vi "Prime calculator.vi"(6 "IR":dbl, 8 "Blue":i16, 9 "Green":i16, 10 "Red":i16, 11 "Clear":i16) -> (0 "B'":dbl, 1 "G'":dbl, 2 "R'":dbl, 3 "C'":dbl)   [LabVIEW 2016, in "AMS TS3472 Light Sensor.lvlib" / "AMS TCS3472.lvclass"]
uses:
  AMS TCS3472.lvclass
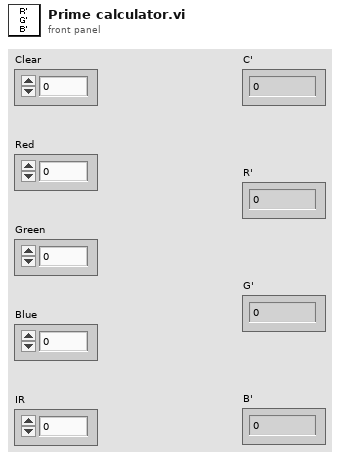
[diagram p1: front panel]
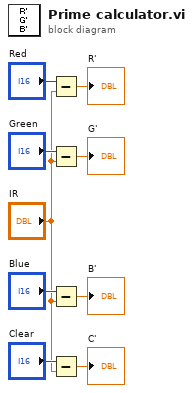
[diagram p0: block diagram]
diagram:
  n1 = Subtract(x="Red", y="IR") -> (x-y=→"R'":dbl)
  n2 = Subtract(x="Green", y="IR") -> (x-y=→"G'":dbl)
  n3 = Subtract(x="Blue", y="IR") -> (x-y=→"B'":dbl)
  n4 = Subtract(x="Clear", y="IR") -> (x-y=→"C'":dbl)
